vi "GFITS_RemoveImNameFmList.vi"(8 "error in (no error)":errorcluster, 10 "Image":string, 11 "Path":path) -> (0 "error out":errorcluster, 2 "answer":string)   [LabVIEW 2016]
uses:
  <vilib>/Utility/config.llb/NI_LVConfig.lvlib
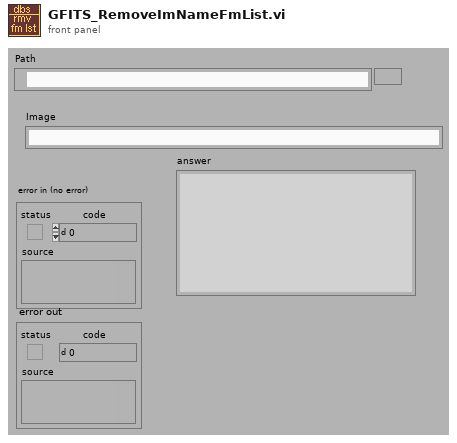
[diagram p1: front panel]
types:
  T1 = typedef "NI_LVConfig.lvlib/Config Data RefNum.ctl" = refnum<k1>
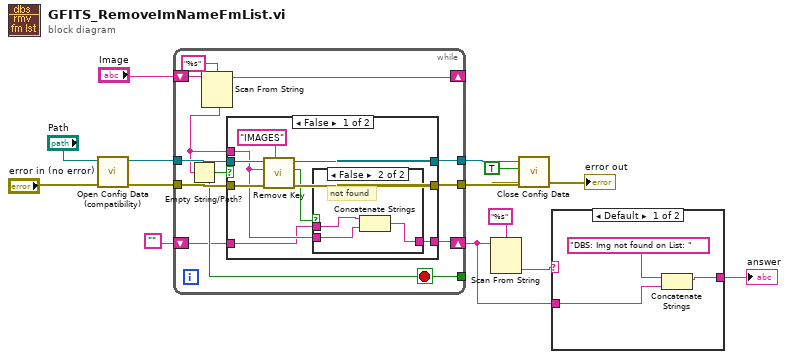
[diagram p0: block diagram]
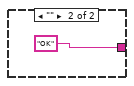
[diagram p4: hidden frame]
diagram:
  n1 = call <vilib>:"Open Config Data (compatibility).vi"("error in (no error)"="error in (no error)", "configuration file path"="Path") -> ("error out"=w10:errorcluster, "refnum"=w13:T1)  [unwired: 7 in, 1 out]
  n2 = while {
    tunnel: w13 -> [w25]
    tunnel: [w24] -> w12
    tunnel: [w23] -> w11
    tunnel: w10 -> [w22]
    shift-right: [w20] -> _
    shift-left: "Image" -> [w21]
    shift-right: [w16] -> w2
    shift-left: "" -> [w15]
    tunnel: [w18] -> _
    stop <- w18 stop-if-true
    n3 = Scan From String(format string="%s", input string=w21) -> (remaining string=w20:string, output 1=w17:string)  [unwired: 2 in, 3 out]
    n4 = Empty String/Path?(string/path=w17) -> (empty?=w18:bool)
    n5 = case shown="False" w18 {
      tunnel: w25 -> [w34 w40]
      tunnel: [w32 w40] -> w24
      tunnel: [w31 w41] -> w23
      tunnel: w22 -> [w30 w41]
      tunnel: w17 -> [w28 _]
      tunnel: [w27 w39] -> w16
      tunnel: w15 -> [w26 w39]
      frame False {
        n6 = call <vilib>:"Remove Key.vi"("section"="IMAGES", "error in (no error)"=w30, "key"=w28, "refnum"=w34) -> ("error out"=w31:errorcluster, "found?"=w29:bool, "refnum out"=w32:T1)  [unwired: 1 in, 4 out]
        n7 = case shown="False" w29 {
          tunnel: w28 -> [_ w38]
          tunnel: [w35 w37] -> w27
          tunnel: w26 -> [w35 w36]
          frame True {
            # "delted"
          }
          frame False {
            # "not found"
            n8 = Concatenate Strings(w36, w38) -> (w37:string)
          }
        }
      }
      frame True {
      }
    }
  }
  n9 = Scan From String(format string="%s", input string=w2) -> (output 1=w3:string)  [unwired: 2 in, 4 out]
  n10 = call <vilib>:"Close Config Data.vi"("error in (no error)"=w11, "write file if changed (T)"=TRUE ("write configuration file? (F)"), "refnum"=w12) -> ("error out"=→"error out":errorcluster)  [unwired: 8 out]
  n11 = case shown="Default" w3 {
    tunnel: [w42 "OK"] -> w7
    tunnel: w2 -> [w43 _]
    frame Default {
      n12 = Concatenate Strings("DBS: Img not found on List: ", w43) -> (w42:string)
    }
    frame "" {
    }
  }
  "answer" <- w7
